vi "Numeric Output Item.vi"(8 "error in (no error)":errorcluster, 9 "Project In":refnum<class "Project.lvclass">, 11 "Output":T2) -> (0 "error out":errorcluster)   [LabVIEW 2015, in "OutputUI.lvclass"]
uses:
  OutputUI.lvclass
  Step/STEP_OUTPUT.ctl
  Step/OUTPUT_DATA_TYPE.ctl
  OUTPUT_CHECK_TYPE.ctl
  Step/OUTPUT_VALUE_TYPE.ctl
  Project.lvclass
  SerializableObject/CONFIGURE_UI_STATE.ctl
  Editor/Editor.lvclass
  Step.lvclass
panel:
  in  "Limit Value Type 2":T1
  in  "Variable Name 2":string(combo)
  in  "Limit Value Type 1":T1
  in  "Variable Name 1":string(combo)
  in  "Upper Limit":dbl
  in  "Low Limit":dbl
  in  "Check":u16(ring)
  out "Type Image":picture
  in  "Output":string
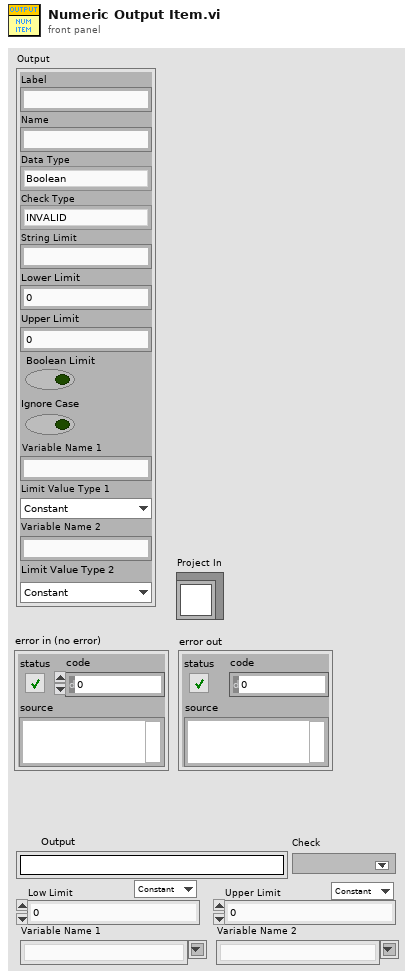
[diagram p1: front panel]
types:
  T1 = typedef "Step.lvclass/OUTPUT_VALUE_TYPE.ctl" = enum16{"Constant", "Variable"}
  T2 = typedef "Step.lvclass/STEP_OUTPUT.ctl" = cluster{"Label":string, "Name":string, "Data Type":T3, "Check Type":T4, "String Limit":string, "Lower Limit":dbl, "Upper Limit":dbl, "Boolean Limit":bool, "Ignore Case":bool, "Variable Name 1":string, "Limit Value Type 1":T1, "Variable Name 2":string, "Limit Value Type 2":T1}
  T3 = typedef "Step.lvclass/OUTPUT_DATA_TYPE.ctl" = enum16{"Boolean", "String", "Numeric", "Other"}
  T4 = typedef "Step.lvclass/OUTPUT_CHECK_TYPE.ctl" = enum16{"INVALID", "DO_NOT_CHECK", "RECORD", "VARIABLE", "EQUAL", "NOT_EQUAL", "STR_CONTAINS", "STR_START_WITH", "STR_END_WITH", "STR_REGEX_MATCH", "NUM_GT", "NUM_LT", "NUM_GE", "NUM_LE", "NUM_RANGE", "NUM_RANGE_BDY"}
  T5 = cluster{"Type Image":refnum<vi>, "Output":refnum<vi>, "Check":refnum<vi>, "Lower Limit":refnum<vi>, "Upper Limit":refnum<vi>, "Variable Name 1":refnum<vi>, "Variable Name 2":refnum<vi>, "Limit Value Type 1":refnum<vi>, "Limit Value Type 2":refnum<vi>}
  T6 = typedef "Editor.lvclass/CONFIGURE_UI_STATE.ctl" = enum16{"UI_LOOP", "INIT", "END", "CHANGE_PANEL"}
  T7 = typedef "LVRectTypeDef.ctl" = cluster{"Left":i16, "Top":i16, "Right":i16, "Bottom":i16}
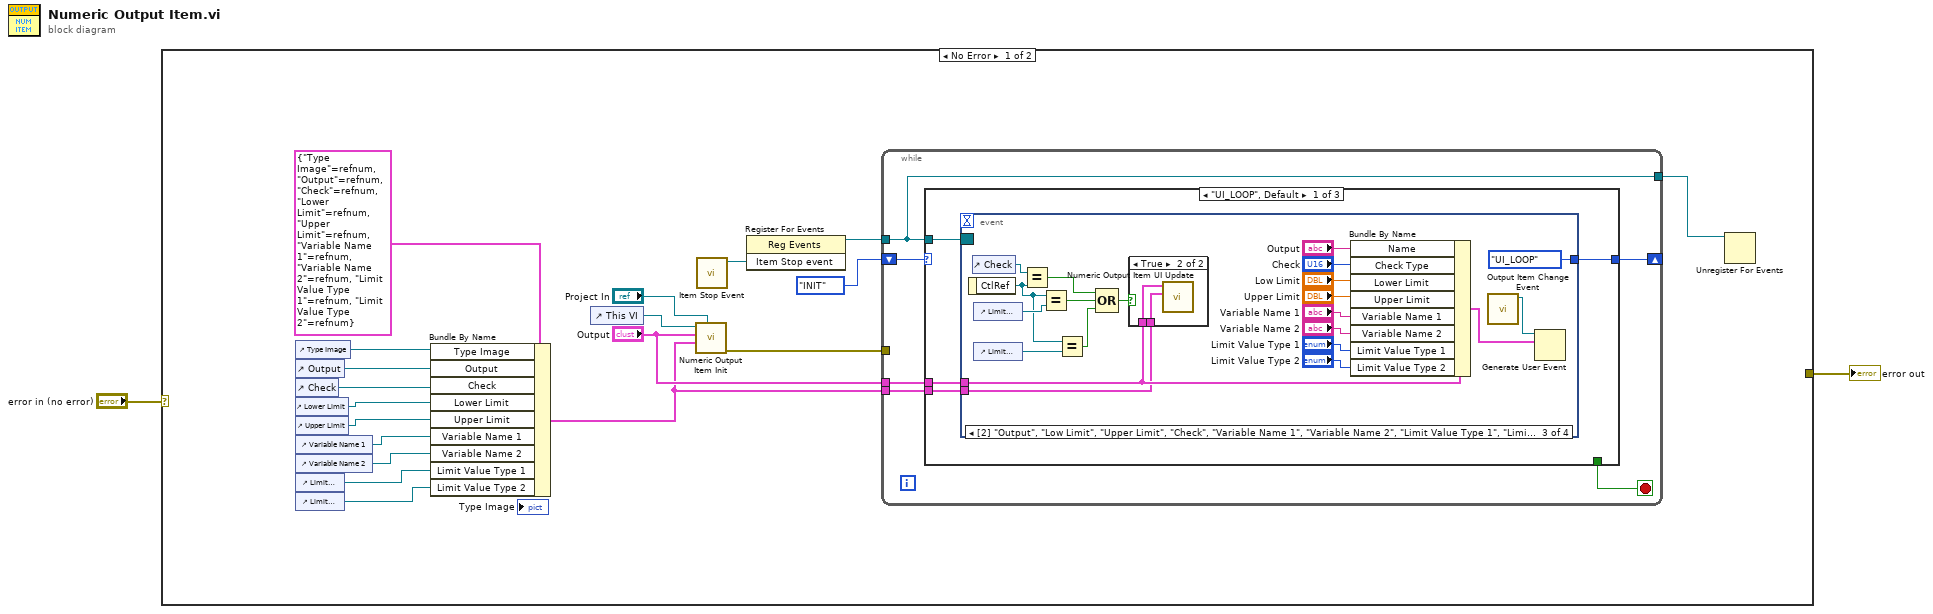
[diagram p0: block diagram]
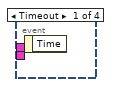
[diagram p2: hidden frame]
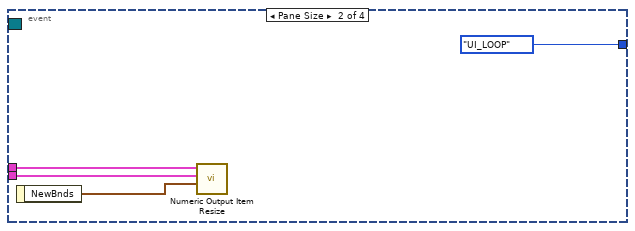
[diagram p3: hidden frame]
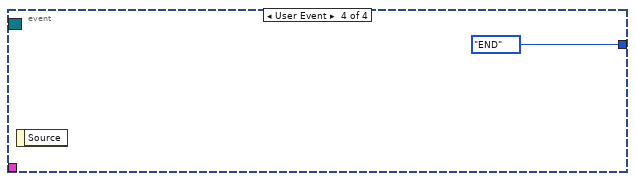
[diagram p5: hidden frame]
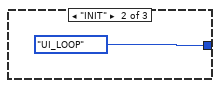
[diagram p6: hidden frame]
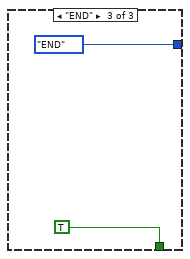
[diagram p7: hidden frame]
diagram:
  n1 = case shown="No Error" "error in (no error)" {
    selector: "error in (no error)" -> [_ w63]
    tunnel: [_ w63] -> w1
    frame No Error {
      n2 = control-ref of="Type Image"() -> (w14:refnum<vi>)
      n3 = control-ref of="Output"() -> (w11:refnum<vi>)
      n4 = control-ref of="Check"() -> (w12:refnum<vi>)
      n5 = control-ref of="Lower Limit"() -> (w9:refnum<vi>)
      n6 = control-ref of="Upper Limit"() -> (w8:refnum<vi>)
      n7 = control-ref of="Variable Name 1"() -> (w7:refnum<vi>)
      n8 = control-ref of="Variable Name 2"() -> (w6:refnum<vi>)
      n9 = control-ref of="Limit Value Type 1"() -> (w5:refnum<vi>)
      n10 = control-ref of="Limit Value Type 2"() -> (w4:refnum<vi>)
      n11 = Bundle By Name(cluster=T5 {"Type Image"=refnum, "Output"=refnum, "Check"=refnum, "Lower Limit"=refnum, "Upper Limit"=refnum, "Variable Name 1"=refnum, "Variable Name 2"=refnum, "Limit Value Type 1"=refnum, "Limit Value Type 2"=refnum} ("UI Elements"), "Type Image"=w14, "Output"=w11, "Check"=w12, "Lower Limit"=w9, "Upper Limit"=w8, "Variable Name 1"=w7, "Variable Name 2"=w6, "Limit Value Type 1"=w5, "Limit Value Type 2"=w4) -> (w3:T5)
      n12 = control-ref of="This VI"() -> (w17:refnum<vi>)
      n13 = call "Numeric Output Item Init.vi"("Project In"="Project In", "Numeric UI Elements"=w3, "Output"="Output", "VI in"=w17) -> ("error out"=w16:errorcluster)  [unwired: 7 in]
      n14 = call "Item Stop Event.vi"() -> ("Item Stop event"=w20:refnum<user-event>)  [unwired: 11 in]
      n15 = register-events(w20) -> (reference out=w19:refnum<event-registration>)  [unwired: 2 in, 1 out]
      n16 = while {
        shift-right: [w26] -> _
        shift-left: CONFIGURE_UI_STATE."INIT" -> [w27]
        tunnel: w19 -> [w24]
        tunnel: [w24] -> w18
        tunnel: w16 -> [_]
        tunnel: "Output" -> [w23]
        tunnel: w3 -> [w22]
        stop <- w25 stop-if-true
        n17 = case shown="\"UI_LOOP\", Default" w27 {
          tunnel: [w31 CONFIGURE_UI_STATE."UI_LOOP" CONFIGURE_UI_STATE."END"] -> w26
          tunnel: [_ _ TRUE] -> w25
          tunnel: w24 -> [w30 _ _]
          tunnel: w23 -> [w29 _ _]
          tunnel: w22 -> [w28 _ _]
          frame "UI_LOOP", Default {
            n18 = event shown="[2] \"Output\", \"Low Limit\", \"Upper Limit\", \"Check\", \"Variable Name 1\", \"Variable Name 2\", \"Limit Value Type 1\", \"Limit Value Type 2\": Value Change" {
              selector: w30 -> [_ _ _ _]
              dyn-events: _ -> [_ _ _ _]
              timeout: _ -> [_ _ _ _]
              tunnel: [_ CONFIGURE_UI_STATE."UI_LOOP" CONFIGURE_UI_STATE."UI_LOOP" CONFIGURE_UI_STATE."END"] -> w31
              tunnel: w29 -> [_ w35 w50 _]
              tunnel: w28 -> [_ w34 w49 _]
              event Timeout {
                n19 = event-data() -> ()  [unwired: 1 in, 1 out]
              }
              event Pane Size {
                n20 = event-data() -> ("NewBnds"=w33:T7)  [unwired: 1 in]
                n21 = call "Numeric Output Item Resize.vi"("NewBnds"=w33, "Numeric UI Elements"=w34, "Output"=w35) -> ()  [unwired: 8 in, 1 out]
              }
              event "Output", "Low Limit", "Upper Limit", "Check", "Variable Name 1", "Variable Name 2": Value Change {
                n22 = event-data() -> ("CtlRef"=w38:refnum<vi>)  [unwired: 1 in]
                n23 = control-ref of="Check"() -> (w51:refnum<vi>)
                n24 = control-ref of="Limit Value Type 1"() -> (w40:refnum<vi>)
                n25 = control-ref of="Limit Value Type 2"() -> (w37:refnum<vi>)
                n26 = Equal?(x=w51, y=w38) -> (x = y?=w41:bool)
                n27 = Equal?(x=w38, y=w40) -> (x = y?=w39:bool)
                n28 = Equal?(x=w38, y=w37) -> (x = y?=w36:bool)
                n29 = Compound Arithmetic op=OR(w41, w39, w36) -> (w42:bool)
                n30 = case shown="True" w42 {
                  tunnel: w50 -> [_ w58]
                  tunnel: w49 -> [_ w57]
                  frame False {
                  }
                  frame True {
                    n31 = call "Numeric Output Item UI Update.vi"("Numeric UI Elements"=w57, "Output"=w58) -> ()  [unwired: 9 in, 1 out]
                  }
                }
                n32 = Bundle By Name(cluster=w50, "Name"="Output", "Check Type"="Check", "Lower Limit"="Low Limit", "Upper Limit"="Upper Limit", "Variable Name 1"="Variable Name 1", "Variable Name 2"="Variable Name 2", "Limit Value Type 1"="Limit Value Type 1", "Limit Value Type 2"="Limit Value Type 2") -> (w52:T2)
                n33 = call "Output Item Change Event.vi"() -> ("Output Value Change Event"=w53:refnum<user-event>)  [unwired: 11 in]
                n34 = Generate User Event(user event=w53, event data cluster=w52) -> ()  [unwired: 2 in, 2 out]
              }
              event User Event {
                n35 = event-data() -> ()  [unwired: 1 in, 1 out]
              }
            }
          }
          frame "INIT" {
          }
          frame "END" {
          }
        }
      }
      n36 = Unregister For Events(event registration refnum=w18) -> ()  [unwired: 1 in, 1 out]
    }
    frame Error {
    }
  }
  "error out" <- w1
